vi "Adam_Ch_Input_Output_ASYNC.vi"(4 "Client Name":string, 6 "Previous Scan Value":dbl format="%.2f", 7 "Value to Output":dbl format="%.2f", 8 "Ch values":dbl[](array[numeric]) format="%.2f", 9 "Scan Period":dbl format="%.2f", 10 "Ch Discription":T1={"Ch Name"="", "Type"="", "Function"=enum."Analogue Input", "Ch State"=enum."On", "Calibration type"="", "A"=0.0, "B"=0.0, "C"=0.0, "D"=0.0, "Comments"="", "Address"={"Main"=0, "Ch."=0, "Sub"=0, "Port Name"=""}, "String"="", "Duty"=65535} {"Duty" format="%016b"; "D" format="%#_5g"; "C" format="%#_5g"; "B" format="%#_5g"; "A" format="%#_5g"}, 11 "Ch names":string[](array[string])) -> (1 "Calibrated units":dbl format="%.2f", 3 "Scan comment":string)   [LabVIEW 2016]
uses:
  ADAM Client/Sub VIs/ADAM Controls/Ch_description_ADAM.ctl
  ADAM Client/Sub VIs/ADAM Controls/Module_type_ADAM.ctl
  ADAM Client/Sub VIs/ADAM Controls/Function_ADAM.ctl
  ADAM Client/Sub VIs/ADAM Controls/Channel_State.ctl
  ADAM Client/Sub VIs/ADAM Controls/Calib_type_ADAM.ctl
  ADAM Client/Sub VIs/ADAM Controls/Address.ctl
  Anemometry/Anemometry Sub Vis/Controls/Serveds.ctl
  ADAM Client/Sub VIs/ADAM Controls/Update_scan_value.ctl
  ADAM_Global.vi
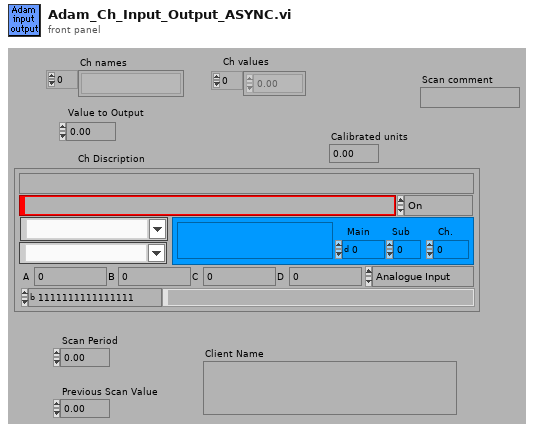
[diagram p1: front panel]
types:
  T1 = typedef "Ch_description_ADAM.ctl" = cluster{"Ch Name":string, "Type":T2, "Function":T3, "Ch State":T4, "Calibration type":T5, "A":dbl, "B":dbl, "C":dbl, "D":dbl, "Comments":string, "Address":T6, "String":string, "Duty":u16}
  T2 = typedef "Module_type_ADAM.ctl" = string
  T3 = typedef "Function_ADAM.ctl" = enum16{"Analogue Input", "Digital Input", "Event counter", "Event rate", "Analogue Output", "Digital Output", "Relay Output"}
  T4 = typedef "Channel_State.ctl" = enum16{"On", "Off", "Always On", "Always Off"}
  T5 = typedef "Calib_type_ADAM.ctl" = string
  T6 = typedef "Address.ctl" = cluster{"Main":i32, "Ch.":i32, "Sub":i32, "Port Name":string}
  T7 = enum16{"Channel Unshared", "Channel Shared by Rig", "Channel Shared by Group"}
  T8 = typedef "Serveds.ctl" = enum16{"Read Global", "Load Global From File"}
  T9 = enum16{"Append to Global", "Read Global then Clear"}
  T10 = typedef "Update_scan_value.ctl" = cluster{"Channel Name":string, "New Value":dbl}
  T11 = typedef "Server_Control.ctl" = cluster{"Channel Name to control":string, "Channel sharing":enum16{"Channel Unshared", "Channel Shared by Rig", "Channel Shared by Group"}, "Default Value":dbl, "Client Array":string[], "Time Stamp":timestamp, "Do Not Reset":bool}
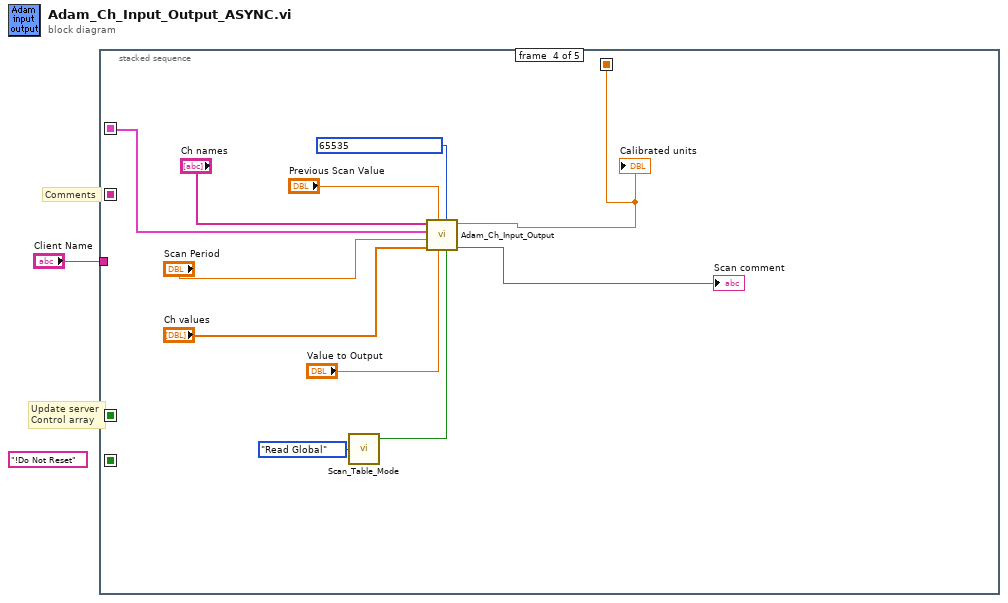
[diagram p0: block diagram]
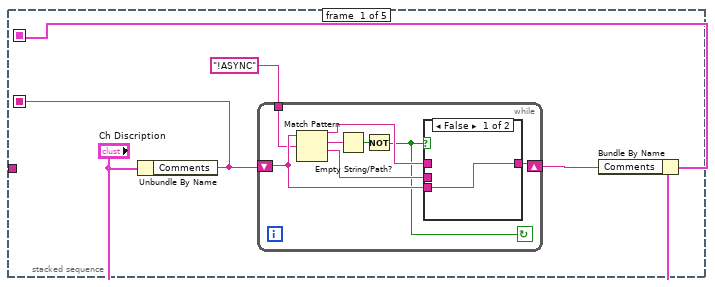
[diagram p2: hidden frame]
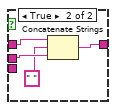
[diagram p3: hidden frame]
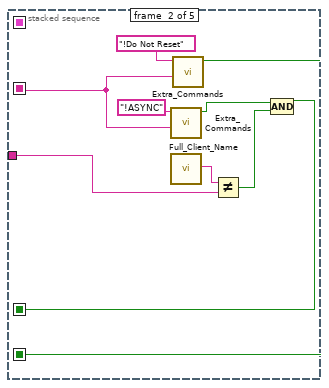
[diagram p4: hidden frame]
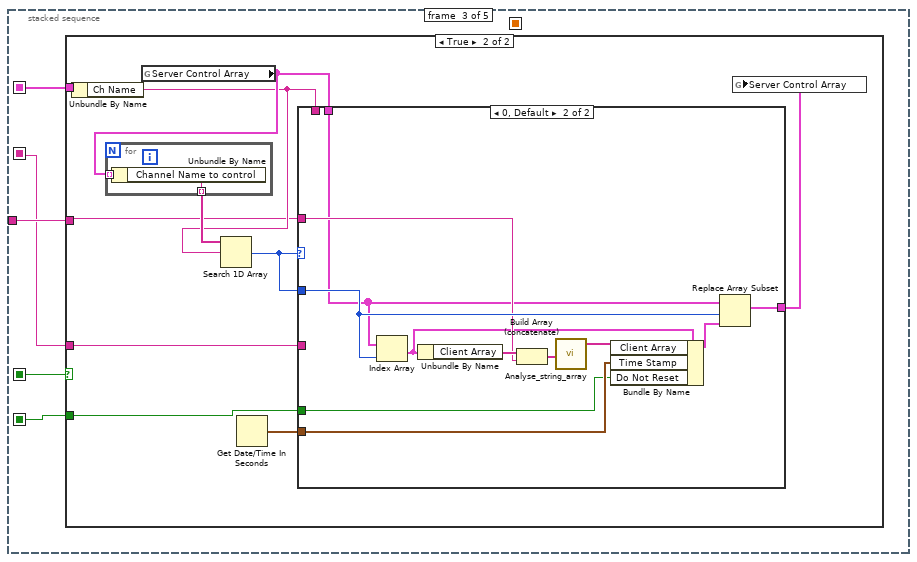
[diagram p5: hidden frame]
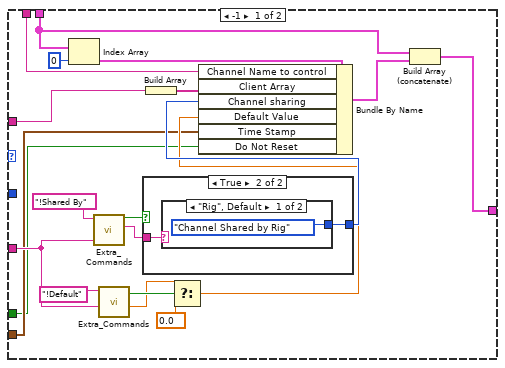
[diagram p7: hidden frame]
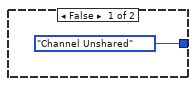
[diagram p8: hidden frame]
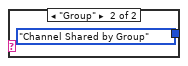
[diagram p9: hidden frame]
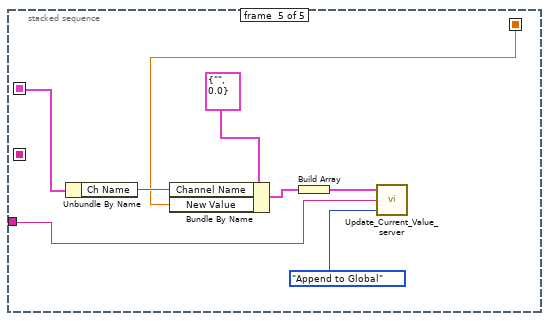
[diagram p10: hidden frame]
diagram:
  (unwired) "!Do Not Reset" ("String to match")
  # "Update server\nControl array"
  # "Comments"
  n1 = stacked-sequence {
    seq-local: [w5 _ _ _ _] -> [_ _ w30 w92 w100]
    seq-local: [_ _ _ w87 _] -> [_ _ _ _ w96]
    seq-local: [w4 _ _ _ _] -> [_ w26 w32 _ _]
    seq-local: [_ w21 _ _ _] -> [_ _ w31 _ _]
    seq-local: [_ w20 _ _ _] -> [_ _ w29 _ _]
    tunnel: "Client Name" -> [_ w23 w33 _ w93]
    frame #0 {
      n2 = Unbundle By Name("Ch Discription") -> ("Comments"=w4:string)
      n3 = while {
        shift-left: w4 -> [w11]
        shift-right: [w12] -> w6
        tunnel: "!ASYNC" ("String to match") -> [w7]
        stop <- w8 continue-if-true
        n4 = Match Pattern(string=w11, regular expression=w7) -> (before substring=w10:string, match substring=w14:string, after substring=w9:string)  [unwired: 2 out]
        n5 = Empty String/Path?(string/path=w14) -> (empty?=w13:bool)
        n6 = Not(x=w13) -> (.not. x?=w8:bool)
        n7 = case shown="False" w8 {
          tunnel: [w15 w18] -> w12
          tunnel: w11 -> [w15 _]
          tunnel: w10 -> [_ w19]
          tunnel: w9 -> [_ w17]
          frame False {
          }
          frame True {
            n8 = Concatenate Strings(w19, " " ("After  Matched string"), w17) -> (w18:string)
          }
        }
      }
      n9 = Bundle By Name(cluster="Ch Discription", "Comments"=w6) -> (w5:T1)
    }
    frame #1 {
      n10 = call "Extra_Commands.vi"("String to Search"=w26, "Command"="!ASYNC" ("String to match")) -> ("Command Found"=w25:bool)  [unwired: 1 in, 4 out]
      n11 = call "Full_Client_Name.vi"() -> ("Client Name"=w24:string)
      n12 = call "Extra_Commands.vi"("String to Search"=w26, "Command"="!Do Not Reset" ("String to match")) -> ("Command Found"=w20:bool)  [unwired: 1 in, 4 out]
      n13 = Not Equal?(x=w24, y=w23) -> (x != y?=w22:bool)
      n14 = Compound Arithmetic op=AND(w25, w22) -> (w21:bool)
    }
    frame #2 {
      n15 = case shown="True" w31 {
        tunnel: w32 -> [_ w42]
        tunnel: w33 -> [_ w35]
        tunnel: w30 -> [_ w43]
        tunnel: w29 -> [_ w34]
        frame False {
        }
        frame True {
          n16 = Unbundle By Name(w43) -> ("Ch Name"=w37:string)
          n17 = global read "ADAM_Global.vi" "Server Control Array"() -> (w40:T11[])
          n18 = for {
            tunnel: w40 -> [w45] mode=indexing
            tunnel: [w44] -> w39 mode=indexing
            n19 = Unbundle By Name(w45) -> ("Channel Name to control"=w44:string)
          }
          n20 = Search 1D Array(1D array=w39, element=w37) -> (index of element=w38:i32)  [unwired: 1 out]
          n21 = Get Date/Time In Seconds() -> (seconds since 1Jan1904=w36:timestamp)
          n22 = case shown="0, Default" w38 {
            tunnel: w38 -> [_ w80]
            tunnel: [w48 w81] -> w41
            tunnel: w35 -> [w52 w78]
            tunnel: w40 -> [w50 w73]
            tunnel: w37 -> [w53 _]
            tunnel: w42 -> [w51 _]
            tunnel: w36 -> [w47 w72]
            tunnel: w34 -> [w46 w71]
            frame -1 {
              n23 = Index Array(array=w50, index=0 ("Index")) -> (element=w54:T11)
              n24 = call "Extra_Commands.vi"("String to Search"=w51, "Command"="!Shared By") -> ("String Value"=w64:string, "Command Found"=w63:bool)  [unwired: 1 in, 3 out]
              n25 = call "Extra_Commands.vi"("String to Search"=w51, "Command"="!Default") -> ("Numeric Value"=w59:dbl, "Command Found"=w60:bool)  [unwired: 1 in, 3 out]
              n26 = case shown="True" w63 {
                tunnel: w64 -> [_ w68]
                tunnel: [T7."Channel Unshared" ("Bundle Element") w67] -> w62
                frame False {
                }
                frame True {
                  n27 = case shown="\"Rig\", Default" w68 {
                    tunnel: [T7."Channel Shared by Rig" ("Bundle Element") T7."Channel Shared by Group" ("Bundle Element")] -> w67
                    frame "Rig", Default {
                    }
                    frame "Group" {
                    }
                  }
                }
              }
              n28 = Build Array(w52) -> (w56:string[])
              n29 = Select(t=w59, s=w60, f=0.0) -> (s? t:f=w57:dbl)
              n30 = Bundle By Name(cluster=w54, "Channel Name to control"=w53, "Client Array"=w56, "Channel sharing"=w62, "Default Value"=w57, "Time Stamp"=w47, "Do Not Reset"=w46) -> (w49:T11)
              n31 = Build Array (concatenate)(w50, w49) -> (w48:T11[])
            }
            frame 0, Default {
              n32 = Index Array(array=w73, index=w80) -> (element=w76:T11)
              n33 = Unbundle By Name(w76) -> ("Client Array"=w79:string[])
              n34 = Build Array (concatenate)(w79, w78) -> (w77:string[])
              n35 = call "Analyse_string_array.vi"("String array"=w77) -> ("Unique strings"=w75:string[])  [unwired: 2 out]
              n36 = Bundle By Name(cluster=w76, "Client Array"=w75, "Time Stamp"=w72, "Do Not Reset"=w71) -> (w74:T11)
              n37 = Replace Array Subset(array=w73, new element=w74, index=w80) -> (w81:T11[])
            }
          }
          n38 = global write "ADAM_Global.vi" "Server Control Array"(w41) -> ()
        }
      }
    }
    frame #3 {
      n39 = call "Scan_Table_Mode.vi"("Mode"=Serveds."Read Global") -> ("Simulate Mode ?"=w82:bool)  [unwired: 2 out]
      n40 = call "Adam_Ch_Input_Output.vi"("Simulate"=w82, "Duty No"=u16 65535, "Value to Output"="Value to Output", "Previuos Scan Value"="Previous Scan Value", "Ch values"="Ch values", "Scan Period"="Scan Period", "Ch Discription"=w92, "Ch names"="Ch names") -> ("Scan comment"=→"Scan comment":string, "Calibrated units"=w87:dbl)  [unwired: 2 out]
      "Calibrated units" <- w87
    }
    frame #4 {
      n41 = Unbundle By Name(w100) -> ("Ch Name"=w98:string)
      n42 = Bundle By Name(cluster=T10 {"Channel Name"="", "New Value"=0.0} ("Update Scan Value Cluster"), "Channel Name"=w98, "New Value"=w96) -> (w97:T10)
      n43 = Build Array(w97) -> (w95:T10[])
      n44 = call "Update_Current_Value_server.vi"("Mode"=T9."Append to Global", "Client HD name"=w93, "Update array in"=w95) -> ()  [unwired: 1 out]
    }
  }
